vi "DashboardIsProgramSaved.vi"(8 "Dashboard":refnum<k24>, 11 "error in":errorcluster) -> (0 "Response":cluster{"Message":string, "Succeed":bool}, 1 "IsSaved":bool, 2 "Name":string, 3 "error out":errorcluster)   [LabVIEW 2022 SP3, in "UnderAutomation.UniversalRobots.lvlib"]
uses:
  UnderAutomation.UniversalRobots.lvlib
  C:/Users/fg/Documents/UniversalRobots.vi/LabVIEW_2024/UnderAutomation.UniversalRobots/lib/UnderAutomation.UniversalRobots.dll
  LabVIEW_2024/UnderAutomation.UniversalRobots/lib/UnderAutomation.UniversalRobots.dll
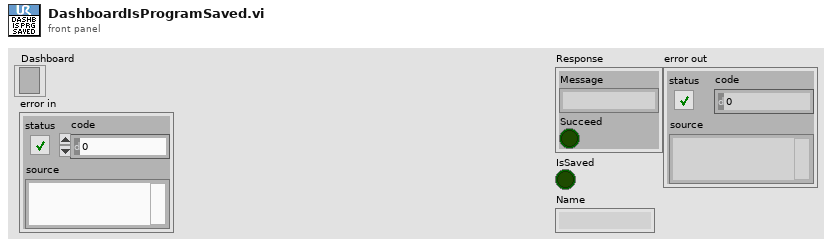
[diagram p1: front panel]
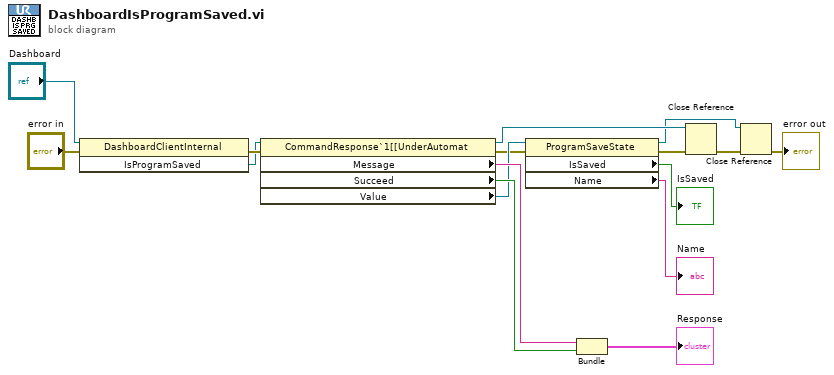
[diagram p0: block diagram]
diagram:
  n1 = invoke class="DashboardClientInternal" method="IsProgramSaved"(reference="Dashboard", error in="error in") -> (error out=w11:errorcluster, "IsProgramSaved"=w7:refnum<k24>)  [unwired: 1 in, 1 out]
  n2 = property class="CommandResponse`1[[UnderAutomat"(reference=w7, error in=w11) -> (reference out=w2:refnum<k24>, error out=w6:errorcluster, "Message"=w15:string, "Succeed"=w14:bool, "Value"=w10:refnum<k24>)
  n3 = property class="ProgramSaveState"(reference=w10, error in=w6) -> (reference out=w1:refnum<k24>, error out=w5:errorcluster, "IsSaved"=→"IsSaved":bool, "Name"=→"Name":string)
  n4 = Bundle("Message"=w15, "Succeed"=w14) -> (→"Response":cluster{"Message":string, "Succeed":bool})  [unwired: 1 in]
  n5 = Close Reference(reference=w2, error in (no error)=w5) -> (error out=w4:errorcluster)
  n6 = Close Reference(reference=w1, error in (no error)=w4) -> (error out=→"error out":errorcluster)
